vi "Write Userinfo.vi"(8 "error in (no error)":errorcluster, 11 "[Data] Userinfo Binary in":refnum<class "[Data] Userinfo Binary.lvclass">) -> (0 "error out":errorcluster, 3 "[Data] Userinfo Binary out":refnum<class "[Data] Userinfo Binary.lvclass">)   [LabVIEW 2020, in "[Data] Userinfo Binary.lvclass"]
uses:
  [Data] Userinfo Binary.lvclass
  [Data] Userinfo Binary.lvclass/[Data] Userinfo Binary.ctl
  <vilib>/YU/YU-Encrypt/AES/AES.lvclass
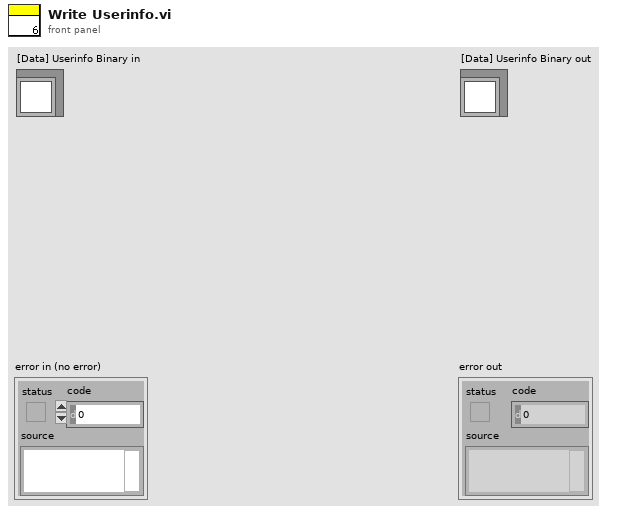
[diagram p1: front panel]
types:
  T1 = enum16{"open", "replace", "create", "open or create", "replace or create", "replace or create with confirmation"}
  T2 = map{string, cluster{"password":string, "department":string, "post":string, "authority":i8, "create time":string, "last login time":string, "remark":string}}
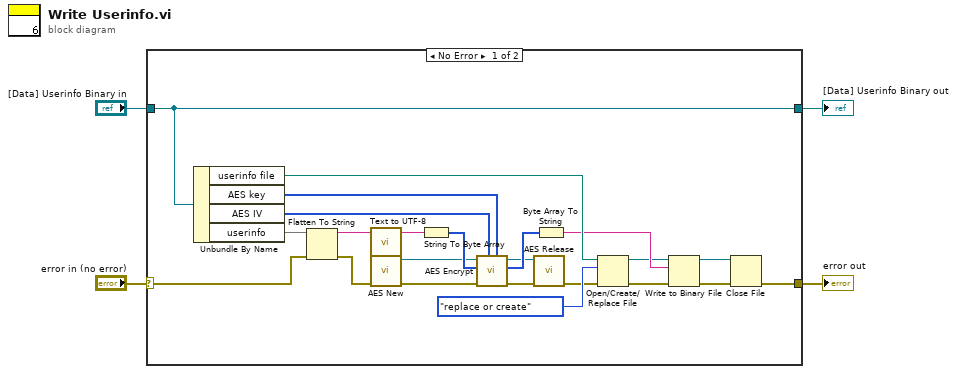
[diagram p0: block diagram]
diagram:
  n1 = case shown="No Error" "error in (no error)" {
    selector: "error in (no error)" -> [w25 w29]
    tunnel: [w8 w29] -> w3
    tunnel: [w27 w28] -> w1
    tunnel: "[Data] Userinfo Binary in" -> [w27 w28]
    frame No Error {
      n2 = Unbundle By Name(w27) -> ("userinfo file"=w15:path, "AES key"=w18:u8[], "AES IV"=w17:u8[], "userinfo"=w26:T2)
      n3 = Flatten To String(anything=w26, error in (no error)=w25) -> (data string=w22:string, error out=w24:errorcluster)  [unwired: 2 in, 1 out]
      n4 = call <vilib>:"Text to UTF-8.vi"("text"=w22) -> ("utf-8 text"=w21:string)  [unwired: 4 in]
      n5 = call <vilib>:"AES New.vi"("error in (no error)"=w24) -> ("error out"=w23:errorcluster, "AES out"=w19:refnum<class "AES.lvclass">)  [unwired: 9 in]
      n6 = String To Byte Array(string=w21) -> (unsigned byte array=w20:u8[])
      n7 = call <vilib>:"AES Encrypt.vi"("Key"=w18, "IV"=w17, "error in (no error)"=w23, "data"=w20, "AES in"=w19) -> ("error out"=w7:errorcluster, "encrypted data"=w16:u8[], "AES out"=w6:refnum<class "AES.lvclass">)  [unwired: 4 in]
      n8 = call <vilib>:"AES Release.vi"("error in (no error)"=w7, "AES in"=w6) -> ("error out"=w5:errorcluster)  [unwired: 9 in]
      n9 = Byte Array To String(unsigned byte array=w16) -> (string=w12:string)
      n10 = Open/Create/Replace File(file path (use dialog)=w15, error in=w5, operation (0:open)=T1."replace or create") -> (refnum out=w11:refnum<file>, error out=w13:errorcluster)  [unwired: 3 in, 1 out]
      n11 = Write to Binary File(file (use dialog)=w11, data=w12, error in=w13) -> (refnum out=w9:refnum<file>, error out=w10:errorcluster)  [unwired: 3 in, 1 out]
      n12 = Close File(refnum=w9, error in=w10) -> (error out=w8:errorcluster)  [unwired: 1 out]
    }
    frame Error {
    }
  }
  "error out" <- w3
  "[Data] Userinfo Binary out" <- w1
